vi "sendValue.vi"(8 "error in (no error)":errorcluster, 10 "data":variant, 11 "performZeroCalib in":refnum<class "performZeroCalib.lvclass">) -> (0 "error out":errorcluster, 2 "function return":i32, 3 "performZeroCalib out":refnum<class "performZeroCalib.lvclass">)   [LabVIEW 2016, in "SALLV_MtAtElectrometer_Messaging.lvlib" / "performZeroCalib.lvclass"]
uses:
  performZeroCalib.lvclass
  ts_sallv_MtAtElectrometer/DataTypes/command_performZeroCalib.ctl
  ts_sallv_MtAtElectrometer/SALLV_MtAtElectrometer.lvlib
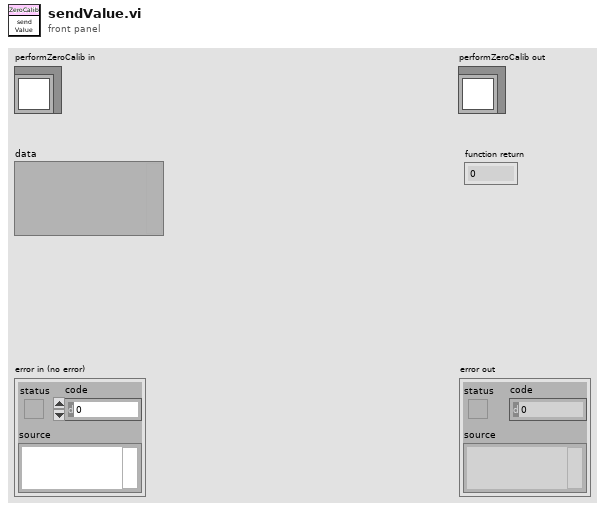
[diagram p1: front panel]
types:
  T1 = typedef "SALLV_MtAtElectrometer.lvlib/command_performZeroCalib.ctl" = cluster{"value":bool}
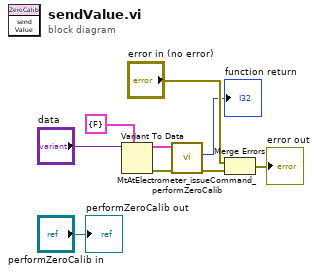
[diagram p0: block diagram]
diagram:
  n1 = Variant To Data(type=T1 {"value"=FALSE} ("command_performZeroCalib_Ctl"), Variant="data") -> (data=w5:T1, error out=w3:errorcluster)  [unwired: 1 in]
  n2 = call "MtAtElectrometer_issueCommand_performZeroCalib.vi"("error in (no error)"=w3, "command_performZeroCalib_Ctl"=w5) -> ("error out"=w2:errorcluster, "function return"=→"function return":i32)  [unwired: 7 in, 1 out]
  n3 = Merge Errors("error in (no error)", w2) -> (→"error out":errorcluster)
  "performZeroCalib out" <- "performZeroCalib in"
